vi "FT10_Fornax Truncate Values.vi"(10 "Auto Set Power Cluster in":T1 {"Power Level" format="%.1f"}) -> (2 "Auto Set Power Cluster out":T1 {"Power Level" format="%.1f"})   [LabVIEW 2015]
doc: "Truncate values greater than 100 and greater than 40 to values divisible by 10 and 5 respectively.\n\nWhy is this needed? -> FT10 power values increase by 5 above 40 and increase by 10 above 100."
uses:
  Controls/Control_Auto Set Power Cluster.ctl
  Controls/Control_Semi-Auto Port.ctl
  Controls/Control_Semi-Auto Mode.ctl
  Controls/Control_Semi-Auto Power Level.ctl
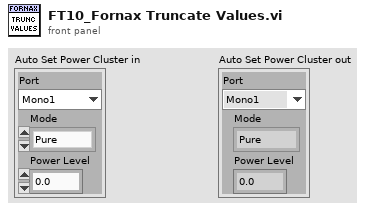
[diagram p1: front panel]
types:
  T1 = typedef "Control_Auto Set Power Cluster.ctl" = cluster{"Port":T2, "Mode":T3, "Power Level":T4}
  T2 = typedef "Control_Semi-Auto Port.ctl" = enum16{"Mono1", "Mono2", "Bipolar", "Ligasure", "Error"}
  T3 = typedef "Control_Semi-Auto Mode.ctl" = enum16{"Pure", "Blend", "Spray", "Fulgerate", "Standard", "Macro", "Precision", "Ligasure", "Error"}
  T4 = typedef "Control_Semi-Auto Power Level.ctl" = dbl
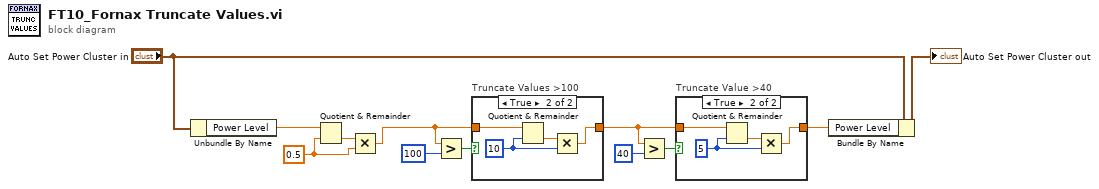
[diagram p0: block diagram]
diagram:
  w3 = 0.5 ("y")
  n1 = Unbundle By Name("Auto Set Power Cluster in") -> ("Power Level"=w2:T4)
  n2 = Quotient & Remainder(x=w2, y=w3) -> (floor(x/y)=w4:T4)  [unwired: 1 out]
  n3 = Multiply(x=w4, y=w3) -> (x*y=w1:T4)
  n4 = Greater?(x=w1, y=100) -> (0:w11:bool)
  n5 = case "Truncate Values >100" shown="True" w11 {
    tunnel: w1 -> [w13 w16]
    tunnel: [w13 w17] -> w8
    frame False {
    }
    frame True {
      w15 = 10 ("y")
      n6 = Quotient & Remainder(x=w16, y=w15) -> (floor(x/y)=w14:T4)  [unwired: 1 out]
      n7 = Multiply(x=w14, y=w15) -> (x*y=w17:T4)
    }
  }
  n8 = Greater?(x=w8, y=40) -> (0:w9:bool)
  n9 = case "Truncate Value >40" shown="True" w9 {
    tunnel: w8 -> [w18 w21]
    tunnel: [w18 w22] -> w5
    frame False {
    }
    frame True {
      w20 = 5 ("y")
      n10 = Quotient & Remainder(x=w21, y=w20) -> (floor(x/y)=w19:T4)  [unwired: 1 out]
      n11 = Multiply(x=w19, y=w20) -> (x*y=w22:T4)
    }
  }
  n12 = Bundle By Name(cluster="Auto Set Power Cluster in", "Power Level"=w5) -> (→"Auto Set Power Cluster out":T1)
